vi "To Variant.vi"(8 "Error In":errorcluster, 11 "2D Int":refnum<class "2D Int.lvclass">) -> (0 "Error Out":errorcluster, 2 "Variant":variant)   [LabVIEW 2017, in "Tree API.lvlib" / "2D Int.lvclass"]
doc: "Dynamic dispatch interface for conversion of Tree Data classes to variant LV data."
uses:
  2D Int.lvclass
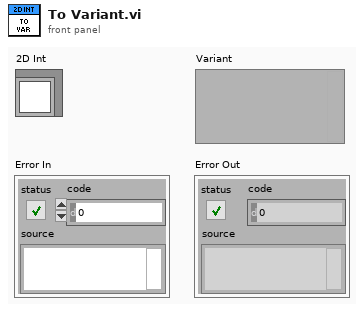
[diagram p1: front panel]
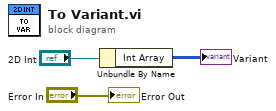
[diagram p0: block diagram]
diagram:
  n1 = Unbundle By Name("2D Int") -> ("Int Array"=→"Variant":i64[][])
  "Error Out" <- "Error In"
